vi "Heila IQ Set V.vi"(8 "error in (no error)":errorcluster, 10 "Voltage Set Point":sgl, 11 "Modbus master in":refnum<class "Modbus Master.lvclass">) -> (0 "error out":errorcluster, 3 "Modbus master out":refnum<class "Modbus Master.lvclass">)   [LabVIEW 2017]
uses:
  <vilib>/Modbus/master/Modbus Master.lvclass
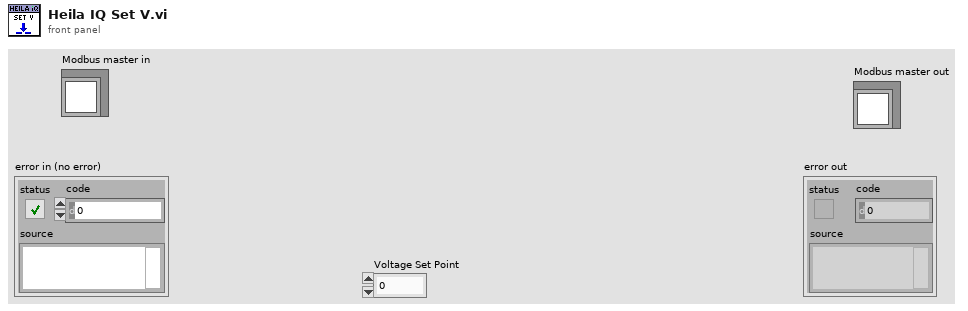
[diagram p1: front panel]
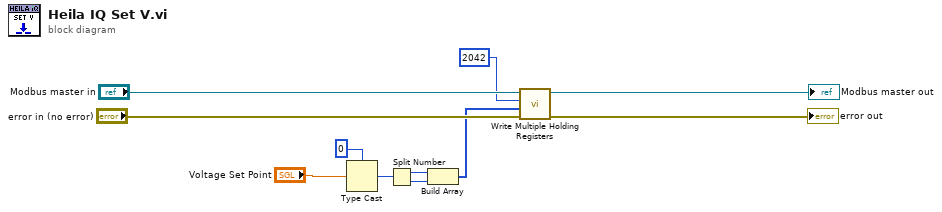
[diagram p0: block diagram]
diagram:
  n1 = Type Cast(type=u32 0, x="Voltage Set Point") -> (*(type *) &x=w6:u32)
  n2 = Split Number(x=w6) -> (hi(x)=w4:u16, lo(x)=w3:u16)
  n3 = Build Array(w4, w3) -> (w2:u16[])
  n4 = call-dynamic "Write Multiple Holding Registers.vi"("error in (no error)"="error in (no error)", "holding register values"=w2, "starting address"=u16 2042, "Modbus master in"="Modbus master in") -> ("error out"=→"error out":errorcluster, "Modbus master out"=→"Modbus master out":refnum<class "Modbus Master.lvclass">)  [unwired: 6 in]
